vi "Simple example.vi"() -> ()   [LabVIEW 2019]
panel:
  out "错误输出":errorcluster
  out "Steps left":i32
  out "Current Position （°）":dbl
  in  "error in (no error)":errorcluster caption="错误输入（无错误）"
  in  "VISA resource name":refnum<visa-resource-name> caption="VISA资源名称"
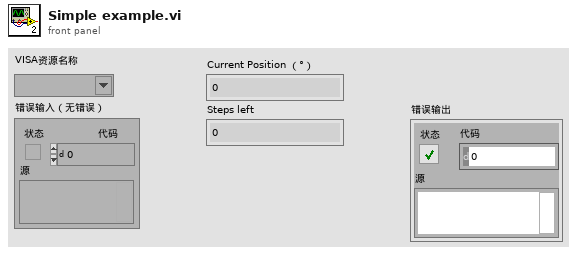
[diagram p1: front panel]
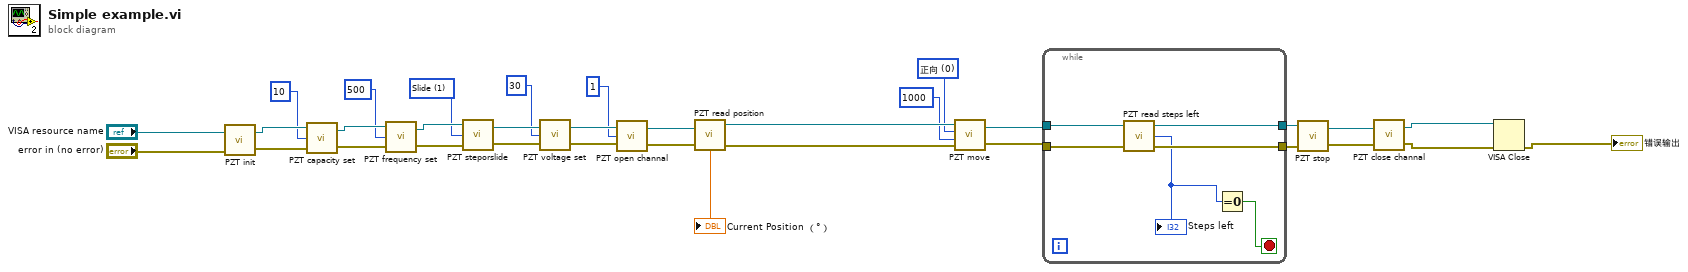
[diagram p0: block diagram]
diagram:
  w10 = u16 0 items=["正向", "反向"] ("移动方向")
  w23 = u16 1 items=["Step", "Slide"] ("运行模式")
  n1 = call "PZT init.vi"("error in (no error)"="error in (no error)", "VISA resource name"="VISA resource name") -> ("错误输出"=w30:errorcluster, "VISA资源名称输出"=w31:refnum<visa-resource-name>)
  n2 = call "PZT capacity set.vi"("error in (no error)"=w30, "电容值（nF）"=10, "VISA resource name"=w31) -> ("错误输出"=w27:errorcluster, "VISA资源名称输出"=w28:refnum<visa-resource-name>)
  n3 = call "PZT frequency set.vi"("error in (no error)"=w27, "频率（Hz）"=500, "VISA resource name"=w28) -> ("错误输出"=w24:errorcluster, "VISA资源名称输出"=w25:refnum<visa-resource-name>)
  n4 = call "PZT steporslide.vi"("error in (no error)"=w24, "运行模式"=w23, "VISA resource name"=w25) -> ("错误输出"=w21:errorcluster, "VISA资源名称输出"=w22:refnum<visa-resource-name>)
  n5 = call "PZT voltage set.vi"("error in (no error)"=w21, "电压值（V）"=30, "VISA resource name"=w22) -> ("错误输出"=w18:errorcluster, "VISA资源名称输出"=w19:refnum<visa-resource-name>)
  n6 = call "PZT open channal.vi"("error in (no error)"=w18, "通道"=1, "VISA resource name"=w19) -> ("错误输出"=w15:errorcluster, "VISA资源名称输出"=w16:refnum<visa-resource-name>)
  n7 = call "PZT read position.vi"("error in (no error)"=w15, "VISA resource name"=w16) -> ("错误输出"=w13:errorcluster, "Current Position （mm  /  °）"=→"Current Position （°）":dbl, "VISA资源名称输出"=w14:refnum<visa-resource-name>)  [unwired: 2 in]
  n8 = call "PZT move.vi"("error in (no error)"=w13, "移动步数"=1000, "移动方向"=w10, "VISA resource name"=w14) -> ("错误输出"=w11:errorcluster, "VISA资源名称输出"=w12:refnum<visa-resource-name>)
  n9 = while {
    tunnel: w12 -> [w39]
    tunnel: [w37] -> w8
    tunnel: w11 -> [w38]
    tunnel: [w36] -> w7
    stop <- w35 stop-if-true
    n10 = call "PZT read steps left.vi"("VISA resource name"=w39, "error in (no error)"=w38) -> ("VISA资源名称输出"=w37:refnum<visa-resource-name>, "Steps left"=w34:i32, "错误输出"=w36:errorcluster)
    "Steps left" <- w34
    n11 = Equal To 0?(x=w34) -> (x = 0?=w35:bool)
  }
  n12 = call "PZT stop.vi"("error in (no error)"=w7, "VISA resource name"=w8) -> ("错误输出"=w5:errorcluster, "VISA资源名称输出"=w6:refnum<visa-resource-name>)
  n13 = call "PZT close channal.vi"("error in (no error)"=w5, "VISA resource name"=w6) -> ("错误输出"=w3:errorcluster, "VISA资源名称输出"=w4:refnum<visa-resource-name>)
  n14 = VISA Close(VISA resource name=w4, error in (no error)=w3) -> (error out=→"错误输出":errorcluster)
